vi "LED Handler.vi"   [LabVIEW 2025]
uses:
  LEDs/Implementation/LEDs Operations.ctl
types:
  T1 = typedef "LEDs Operations.ctl" = enum16{"Reserve", "Read Current", "Immediate", "No Game Data", "Game Period", "Set Color", "Knight Rider"}
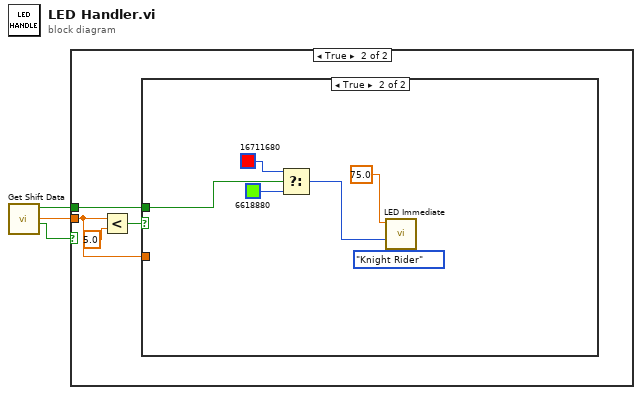
[diagram p0: block diagram]
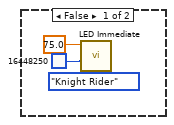
[diagram p2: hidden frame]
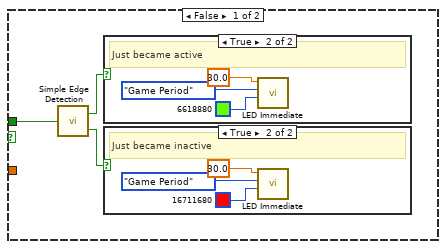
[diagram p3: hidden frame]
diagram:
  n1 = call "Get Shift Data.vi"() -> ("Game Data Received"=w1:bool, "Time Until Next Change"=w2:dbl, "Current Shift Active?"=w3:bool)  [unwired: 9 in]
  n2 = case shown="True" w1 {
    tunnel: w3 -> [_ w10]
    tunnel: w2 -> [_ w7]
    frame False {
      n3 = call "LED Immediate.vi"("Color Box"=u32 16448250, "Operation"=LEDs_Operations."Knight Rider", "Sine Wave"=75.0) -> ()  [unwired: 8 in, 1 out]
    }
    frame True {
      n4 = Less?(x=w7, y=5.0) -> (x < y?=w8:bool)
      n5 = case shown="True" w8 {
        tunnel: w10 -> [w13 w24]
        tunnel: w7 -> [_ _]
        frame False {
          n6 = call "Simple Edge Detection.vi"("In"=w13) -> ("Rising Edge"=w12:bool, "Falling Edge"=w11:bool)
          n7 = case shown="True" w12 {
            frame False {
            }
            frame True {
              # "Just became active"
              n8 = call "LED Immediate.vi"("Color Box"=u32 6618880, "Operation"=LEDs_Operations."Game Period", "Sine Wave"=30.0) -> ()  [unwired: 8 in, 1 out]
            }
          }
          n9 = case shown="True" w11 {
            frame False {
            }
            frame True {
              # "Just became inactive"
              n10 = call "LED Immediate.vi"("Color Box"=u32 16711680, "Operation"=LEDs_Operations."Game Period", "Sine Wave"=30.0) -> ()  [unwired: 8 in, 1 out]
            }
          }
        }
        frame True {
          n11 = Select(t=u32 16711680 ("Color Box"), s=w24, f=u32 6618880 ("Color Box")) -> (s? t:f=w21:u32)
          n12 = call "LED Immediate.vi"("Color Box"=w21, "Operation"=LEDs_Operations."Knight Rider", "Sine Wave"=75.0) -> ()  [unwired: 8 in, 1 out]
        }
      }
    }
  }
